vi "Error Query.vi"(8 "error in (no error)":errorcluster, 11 "VISA resource name":refnum<visa-resource-name>) -> (0 "error out":errorcluster, 1 "Error Message":string, 2 "Error Code":i32[](array[numeric]), 3 "VISA resource name out":refnum<visa-resource-name>)   [LabVIEW 2012, in "Fluke 8508.lvlib"]
doc: "This VI queries the instrument for any errors in the instrument's error queue. It will continue to read errors until all errors have been read from the instrument. Any errors will be returned in the Error Out cluster.\n\nNote:\nThis VI is called automatically by most driver VIs so it is not usually necessary to call this in an application."
uses:
  Fluke 8508.lvlib
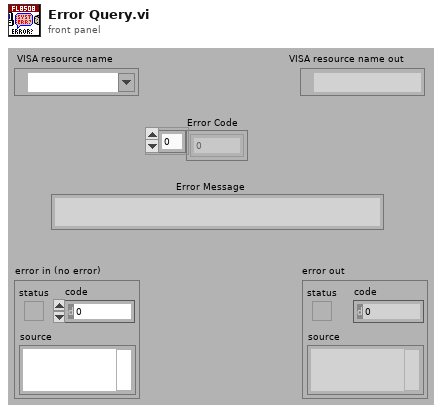
[diagram p1: front panel]
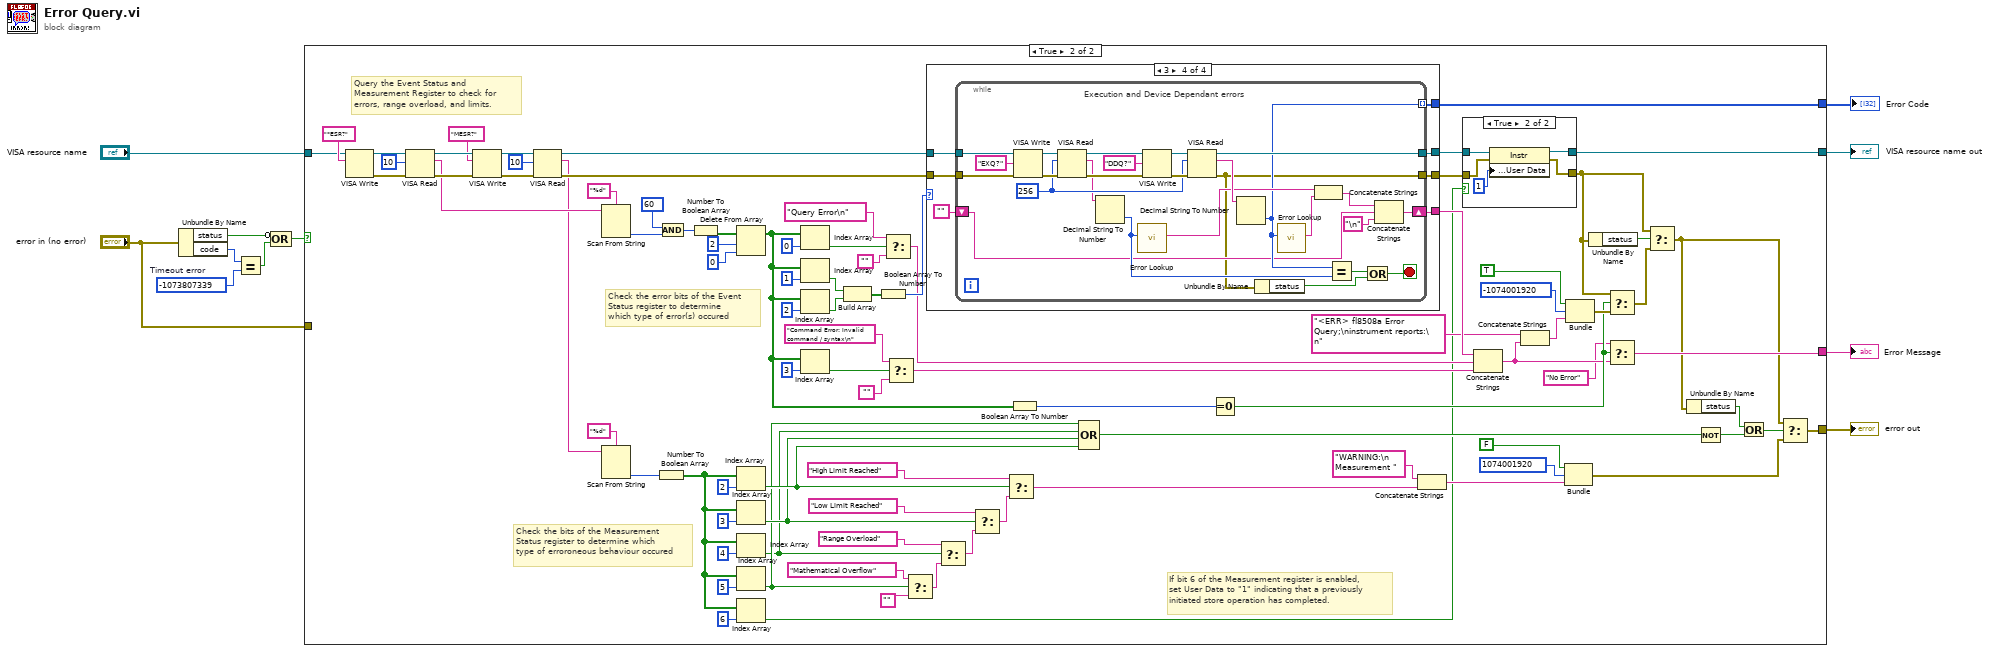
[diagram p0: block diagram]
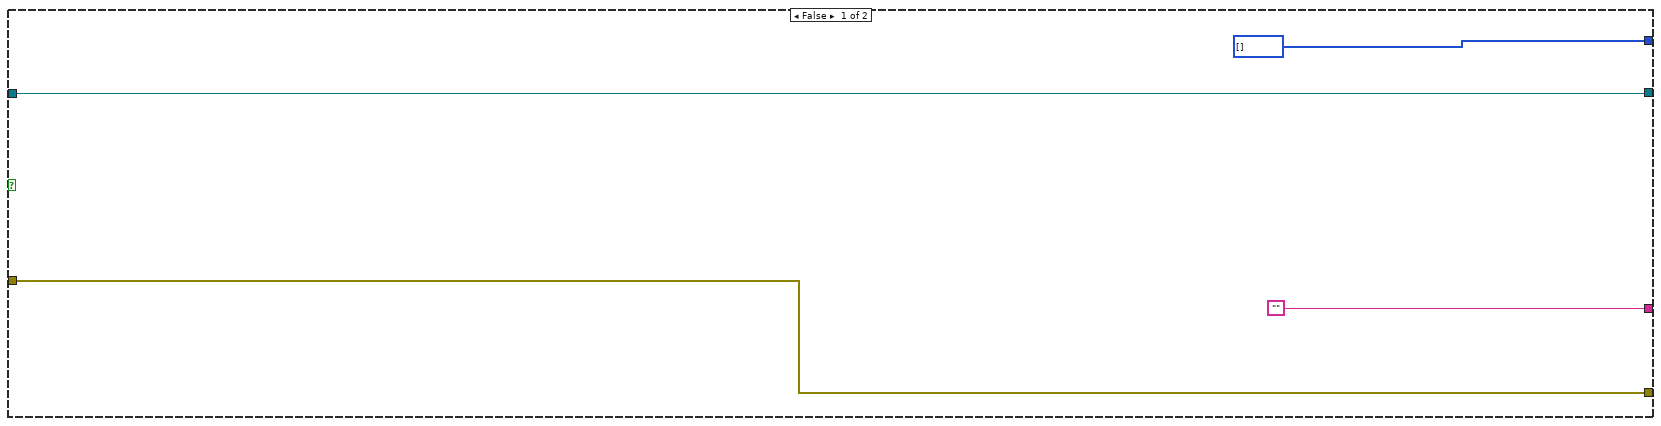
[diagram p2: hidden frame]
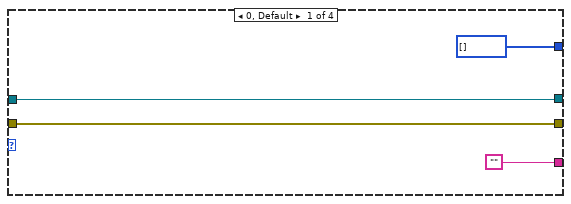
[diagram p4: hidden frame]
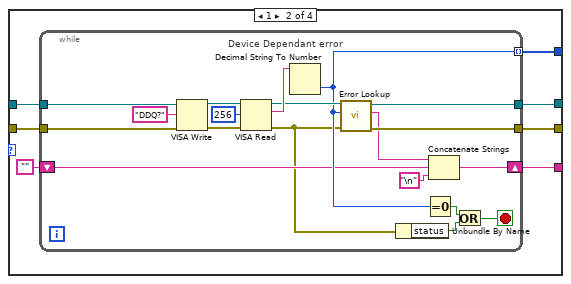
[diagram p5: hidden frame]
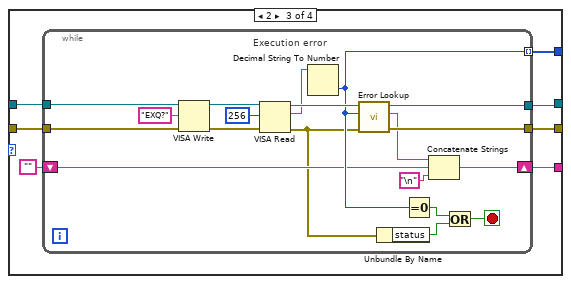
[diagram p6: hidden frame]
diagram:
  w2 = -1073807339  # Timeout error
  n1 = Unbundle By Name("error in (no error)") -> ("status"=w6:bool, "code"=w4:i32)
  n2 = Equal?(x=w4, y=w2) -> (x = y?=w5:bool)
  n3 = Compound Arithmetic op=OR(invert w6, w5) -> (w3:bool)
  n4 = case shown="True" w3 {
    tunnel: "VISA resource name" -> [w13 w75]
    tunnel: ["" w64] -> w10
    tunnel: [i32[] [] w74] -> w9
    tunnel: [w12 w22] -> w8
    tunnel: [w13 w19] -> w7
    tunnel: "error in (no error)" -> [w12 _]
    frame False {
    }
    frame True {
      # "If bit 6 of the Measurement register is enabled, set User Data to \"1\" indicating that a previously initiated store operation has completed."
      # "Check the bits of the Measurement Status register to determine which type of erroroneous behaviour occured"
      # "Check the error bits of the Event Status register to determine which type of error(s) occured"
      # "Query the Event Status and Measurement Register to check for errors, range overload, and limits."
      n5 = VISA Write(VISA resource name=w75, write buffer="*ESR?") -> (VISA resource name out=w84:refnum<visa-resource-name>, error out=w83:errorcluster)  [unwired: 1 in, 1 out]
      n6 = VISA Read(VISA resource name=w84, byte count=10, error in (no error)=w83) -> (VISA resource name out=w61:refnum<visa-resource-name>, read buffer=w56:string, error out=w60:errorcluster)  [unwired: 1 out]
      n7 = VISA Write(VISA resource name=w61, write buffer="MESR?", error in (no error)=w60) -> (VISA resource name out=w62:refnum<visa-resource-name>, error out=w58:errorcluster)  [unwired: 1 out]
      n8 = VISA Read(VISA resource name=w62, byte count=10, error in (no error)=w58) -> (VISA resource name out=w55:refnum<visa-resource-name>, read buffer=w52:string, error out=w54:errorcluster)  [unwired: 1 out]
      n9 = Scan From String(format string="%d", input string=w56) -> (output 1=w73:i32)  [unwired: 3 in, 3 out]
      n10 = Scan From String(format string="%d", input string=w52) -> (output 1=w51:i32)  [unwired: 3 in, 3 out]
      n11 = Number To Boolean Array(number=w51) -> (Boolean array=w38:bool[])
      n12 = And(x=60, y=w73) -> (x .and. y?=w100:i32)
      n13 = Number To Boolean Array(number=w100) -> (Boolean array=w103:bool[])
      n14 = Delete From Array(array=w103, length=2, index=0) -> (array with subset deleted=w70:bool[])  [unwired: 1 out]
      n15 = Index Array(array=w38, index=2) -> (element=w36:bool)
      n16 = Index Array(array=w38, index=3) -> (element=w35:bool)
      n17 = Index Array(array=w38, index=4) -> (element=w33:bool)
      n18 = Index Array(array=w38, index=5) -> (element=w34:bool)
      n19 = Index Array(array=w38, index=6) -> (element=w16:bool)
      n20 = Index Array(array=w70, index=0) -> (element=w91:bool)
      n21 = Index Array(array=w70, index=1) -> (element=w95:bool)
      n22 = Index Array(array=w70, index=2) -> (element=w94:bool)
      n23 = Index Array(array=w70, index=3) -> (element=w88:bool)
      n24 = Build Array(w95, w94) -> (w93:bool[])
      n25 = Boolean Array To Number(Boolean array=w93) -> (number=w92:u32)
      n26 = Select(t="Query Error\n", s=w91, f="") -> (s? t:f=w80:string)
      n27 = Select(t="Command Error: Invalid  command / syntax\n", s=w88, f="") -> (s? t:f=w79:string)
      n28 = Select(t="Mathematical Overflow" ("write buffer"), s=w34, f="") -> (s? t:f=w46:string)
      n29 = case shown="3" w92 {
        tunnel: w55 -> [w116 w123 w149 w175]
        tunnel: w54 -> [w115 w122 w148 w174]
        tunnel: [w116 w121 w147 w172] -> w20
        tunnel: [w115 w120 w146 w173] -> w18
        tunnel: ["" ("Error Message") w119 w144 w171] -> w81
        tunnel: [i32[] [] w118 w145 w170] -> w74
        frame 0, Default {
        }
        frame 1 {
          n30 = while {
            tunnel: w123 -> [w138]
            tunnel: w122 -> [w137]
            tunnel: [w134] -> w121
            tunnel: [w133] -> w120
            tunnel: [w132] -> w118 mode=indexing
            shift-right: [w129] -> w119
            shift-left: "" -> [w128]
            stop <- w124 stop-if-true
            # "Device Dependant error"
            n31 = VISA Write(VISA resource name=w138, write buffer="DDQ?", error in (no error)=w137) -> (VISA resource name out=w141:refnum<visa-resource-name>, error out=w140:errorcluster)  [unwired: 1 out]
            n32 = VISA Read(VISA resource name=w141, byte count=u32 256, error in (no error)=w140) -> (VISA resource name out=w135:refnum<visa-resource-name>, read buffer=w136:string, error out=w127:errorcluster)  [unwired: 1 out]
            n33 = Decimal String To Number(string=w136) -> (number=w132:i32)  [unwired: 2 in, 1 out]
            n34 = call "Error Lookup.vi"("error in (no error)"=w127, "Error code"=w132, "VISA resource name"=w135) -> ("error out"=w133:errorcluster, "Error Message"=w130:string, "VISA resource name out"=w134:refnum<visa-resource-name>)  [unwired: 6 in]
            n35 = Unbundle By Name(w127) -> ("status"=w125:bool)
            n36 = Equal To 0?(x=w132) -> (x = 0?=w126:bool)
            n37 = Concatenate Strings(w130, w128, "\n" ("string")) -> (w129:string)
            n38 = Or(x=w126, y=w125) -> (x .or. y?=w124:bool)
          }
        }
        frame 2 {
          n39 = while {
            tunnel: w149 -> [w168]
            tunnel: w148 -> [w167]
            tunnel: [w160] -> w147
            tunnel: [w159] -> w146
            tunnel: [w158] -> w145 mode=indexing
            shift-right: [w157] -> w144
            shift-left: "" -> [w155]
            stop <- w154 stop-if-true
            # "Execution error"
            n40 = VISA Write(VISA resource name=w168, write buffer="EXQ?", error in (no error)=w167) -> (VISA resource name out=w166:refnum<visa-resource-name>, error out=w165:errorcluster)  [unwired: 1 out]
            n41 = VISA Read(VISA resource name=w166, byte count=u32 256, error in (no error)=w165) -> (VISA resource name out=w162:refnum<visa-resource-name>, read buffer=w161:string, error out=w152:errorcluster)  [unwired: 1 out]
            n42 = Decimal String To Number(string=w161) -> (number=w158:i32)  [unwired: 2 in, 1 out]
            n43 = call "Error Lookup.vi"("error in (no error)"=w152, "Error code"=w158, "VISA resource name"=w162) -> ("error out"=w159:errorcluster, "Error Message"=w156:string, "VISA resource name out"=w160:refnum<visa-resource-name>)  [unwired: 6 in]
            n44 = Unbundle By Name(w152) -> ("status"=w151:bool)
            n45 = Equal To 0?(x=w158) -> (x = 0?=w153:bool)
            n46 = Concatenate Strings(w156, w155, "\n" ("string")) -> (w157:string)
            n47 = Or(x=w153, y=w151) -> (x .or. y?=w154:bool)
          }
        }
        frame 3 {
          n48 = while {
            tunnel: w175 -> [w201]
            tunnel: w174 -> [w200]
            tunnel: [w177] -> w173
            tunnel: [w188] -> w172
            tunnel: [w184] -> w170 mode=indexing
            shift-right: [w182] -> w171
            shift-left: "" -> [w180]
            stop <- w179 stop-if-true
            w191 = u32 256 ("byte count")
            # "Execution and Device Dependant errors"
            n49 = VISA Write(VISA resource name=w201, write buffer="EXQ?", error in (no error)=w200) -> (VISA resource name out=w199:refnum<visa-resource-name>, error out=w198:errorcluster)  [unwired: 1 out]
            n50 = VISA Read(VISA resource name=w199, byte count=w191, error in (no error)=w198) -> (VISA resource name out=w197:refnum<visa-resource-name>, read buffer=w190:string, error out=w196:errorcluster)  [unwired: 1 out]
            n51 = Decimal String To Number(string=w190) -> (number=w185:i32)  [unwired: 2 in, 1 out]
            n52 = call "Error Lookup.vi"("Error code"=w185) -> ("Error Message"=w187:string)  [unwired: 8 in, 2 out]
            n53 = VISA Write(VISA resource name=w197, write buffer="DDQ?", error in (no error)=w196) -> (VISA resource name out=w195:refnum<visa-resource-name>, error out=w194:errorcluster)  [unwired: 1 out]
            n54 = VISA Read(VISA resource name=w195, byte count=w191, error in (no error)=w194) -> (VISA resource name out=w188:refnum<visa-resource-name>, read buffer=w189:string, error out=w177:errorcluster)  [unwired: 1 out]
            n55 = Decimal String To Number(string=w189) -> (number=w184:i32)  [unwired: 2 in, 1 out]
            n56 = Unbundle By Name(w177) -> ("status"=w176:bool)
            n57 = call "Error Lookup.vi"("Error code"=w184) -> ("Error Message"=w186:string)  [unwired: 8 in, 2 out]
            n58 = Concatenate Strings(w187, w186) -> (w181:string)
            n59 = Equal?(x=w184, y=w185) -> (x = y?=w178:bool)
            n60 = Or(x=w178, y=w176) -> (x .or. y?=w179:bool)
            n61 = Concatenate Strings(w181, w180, "\n" ("string")) -> (w182:string)
          }
        }
      }
      n62 = Select(t="Range Overload" ("write buffer"), s=w33, f=w46) -> (s? t:f=w44:string)
      n63 = Select(t="Low Limit Reached" ("write buffer"), s=w35, f=w44) -> (s? t:f=w41:string)
      n64 = Select(t="High Limit Reached" ("write buffer"), s=w36, f=w41) -> (s? t:f=w29:string)
      n65 = Boolean Array To Number(Boolean array=w70) -> (number=w69:u32)
      n66 = Compound Arithmetic op=OR(w34, w33, w35, w36) -> (w24:bool)
      n67 = Equal To 0?(x=w69) -> (x = 0?=w66:bool)
      n68 = Concatenate Strings("WARNING:\n Measurement " ("string"), w29) -> (w32:string)
      n69 = case shown="True" w16 {
        tunnel: [w107 w111] -> w19
        tunnel: w20 -> [w107 w112]
        tunnel: [w106 w109] -> w17
        tunnel: w18 -> [w106 w110]
        frame False {
        }
        frame True {
          n70 = property class="Instr"(reference=w112, error in=w110, "General Settings:User Data"=u32 1) -> (reference out=w111:refnum<visa-resource-name>, error out=w109:errorcluster)
        }
      }
      n71 = Concatenate Strings(w81, w80, w79) -> (w65:string)
      n72 = Concatenate Strings("<ERR> fl8508a Error Query;\ninstrument reports:\n" ("Source"), w65) -> (w67:string)
      n73 = Bundle(FALSE, 1074001920, w32) -> (w26:errorcluster)  [unwired: 1 in]
      n74 = Bundle(TRUE, -1074001920, w67) -> (w72:errorcluster)  [unwired: 1 in]
      n75 = Unbundle By Name(w17) -> ("status"=w76:bool)
      n76 = Select(t=w17, s=w66, f=w72) -> (s? t:f=w71:errorcluster)
      n77 = Select(t="No Error", s=w66, f=w65) -> (s? t:f=w64:string)
      n78 = Select(t=w17, s=w76, f=w71) -> (s? t:f=w21:errorcluster)
      n79 = Unbundle By Name(w21) -> ("status"=w25:bool)
      n80 = Not(x=w24) -> (.not. x?=w23:bool)
      n81 = Or(x=w25, y=w23) -> (x .or. y?=w27:bool)
      n82 = Select(t=w21, s=w27, f=w26) -> (s? t:f=w22:errorcluster)
    }
  }
  "VISA resource name out" <- w7
  "error out" <- w8
  "Error Message" <- w10
  "Error Code" <- w9
